vi "test.vi"() -> ()   [LabVIEW 2020]
uses:
  <userlib>/cDaq/cDaq.lvlib
panel:
  out "handle":u32
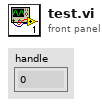
[diagram p1: front panel]
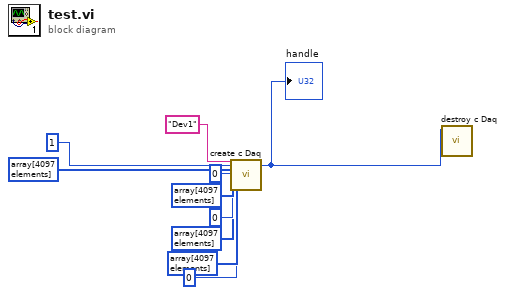
[diagram p0: block diagram]
diagram:
  n1 = call <userlib>:"create c Daq .vi"("device"="Dev1", "analog_count"=1, "analog_io_id"=i32[] array[4097 elements], "digital_count"=0, "digital_io_id"=i32[] array[4097 elements], "analog_co_count"=0, "analog_co_io_id"=i32[] array[4097 elements], "digital_co_count"=0, "digital_co_io_id"=i32[] array[4097 elements]) -> ("function return"=w7:u32)  [unwired: 13 in, 5 out]
  "handle" <- w7
  n2 = call <userlib>:"destroy c Daq .vi"("handle"=w7) -> ()  [unwired: 9 in, 2 out]
